vi "Object Tracking V2.vi"() -> ()   [LabVIEW 2012]
uses:
  <vilib>/userdefined/High Color/IMAQdx.ctl
  <vilib>/vision/Pattern Matching.llb/IMAQ Curve Parameters.ctl
  <vilib>/vision/driver/IMAQdx.llb/IMAQdx Buffer Number Mode.ctl
  <vilib>/vision/driver/NI_Vision_Acquisition_Software.lvlib
  <vilib>/vision/NI_Vision_Development_Module.lvlib
panel:
  in  "Match Type":enum16{"Geometric Matching", "Pattern Matching"}(ring)=enum."Pattern Matching"
  in  "Match":bool
  out "Matches":T1(array[cluster]) {"Bounding Box"."y" format="%.2f"; "Bounding Box"."x" format="%.2f"; "Position"."y" format="%.2f"; "Position"."x" format="%.2f"; "Score" format="%.2f"; "Scale" format="%.2f"; "Angle" format="%.2f"}
  in  "Learn":bool
  in  "Snap Frame":bool
  in  "Camera Name":T2="cam0"
  in  "Stop Button":bool
  in  "Geometric Match Mode":T3={"Rotation"=TRUE, "Scale"=FALSE, "Occlusion"=FALSE, "Reserved"=FALSE, "Reserved"=FALSE, "Reserved"=FALSE}
  in  "Pattern Match Mode":u16(ring)=1 items=["Shift Invariant", "Rotation Invariant"]
  in  "Minimum Score":sgl=600.0
  in  "Nb of Matches":i32=1
  in  "Subpixel Accuracy":bool
  in  "Minimum Contrast":i32=10
  in  "Curve Parameters":T4={"Extraction Mode"=0, "Edge Threshold"=75, "Edge Filter Size"=1, "Min Length"=25, "Row Search Step Size"=15, "Col Search Step Size"=15, "Max Endpoint Gap"=10, "Closed"=FALSE, "Subpixel"=FALSE} {"Extraction Mode" items=["Normal", "Uniform Regions"]; "Edge Filter Size" items=["Fine", "Normal", "Contour Tracing"]; "Max Endpoint Gap" min=0; "Col Search Step Size" min=1 max=255 step=1; "Row Search Step Size" min=1 max=255 step=1; "Min Length" min=0; "Edge Threshold" min=1 max=350 step=1}
  out "Template":T5(plugin-control)
  out "Snap Image":T5(plugin-control)
  out "Image Out":T5(plugin-control)
  # "1. Run the VI\n\n2. Click \"Snap Frame\" (make sure the object that you want to track\nit in the image at the time you snap the frame\n\n3. Use the mouse to select that object that you wish to track. This is done in the bottow left frame,\n\n4. Click \"Learn\" (This area is not saved at the new template image as seen in the bottom right frame)\n\n5. Click \"Match\" the program will then look for the template image and display the resutls with a red box."
  # "1."
  # "2."
  # "3."
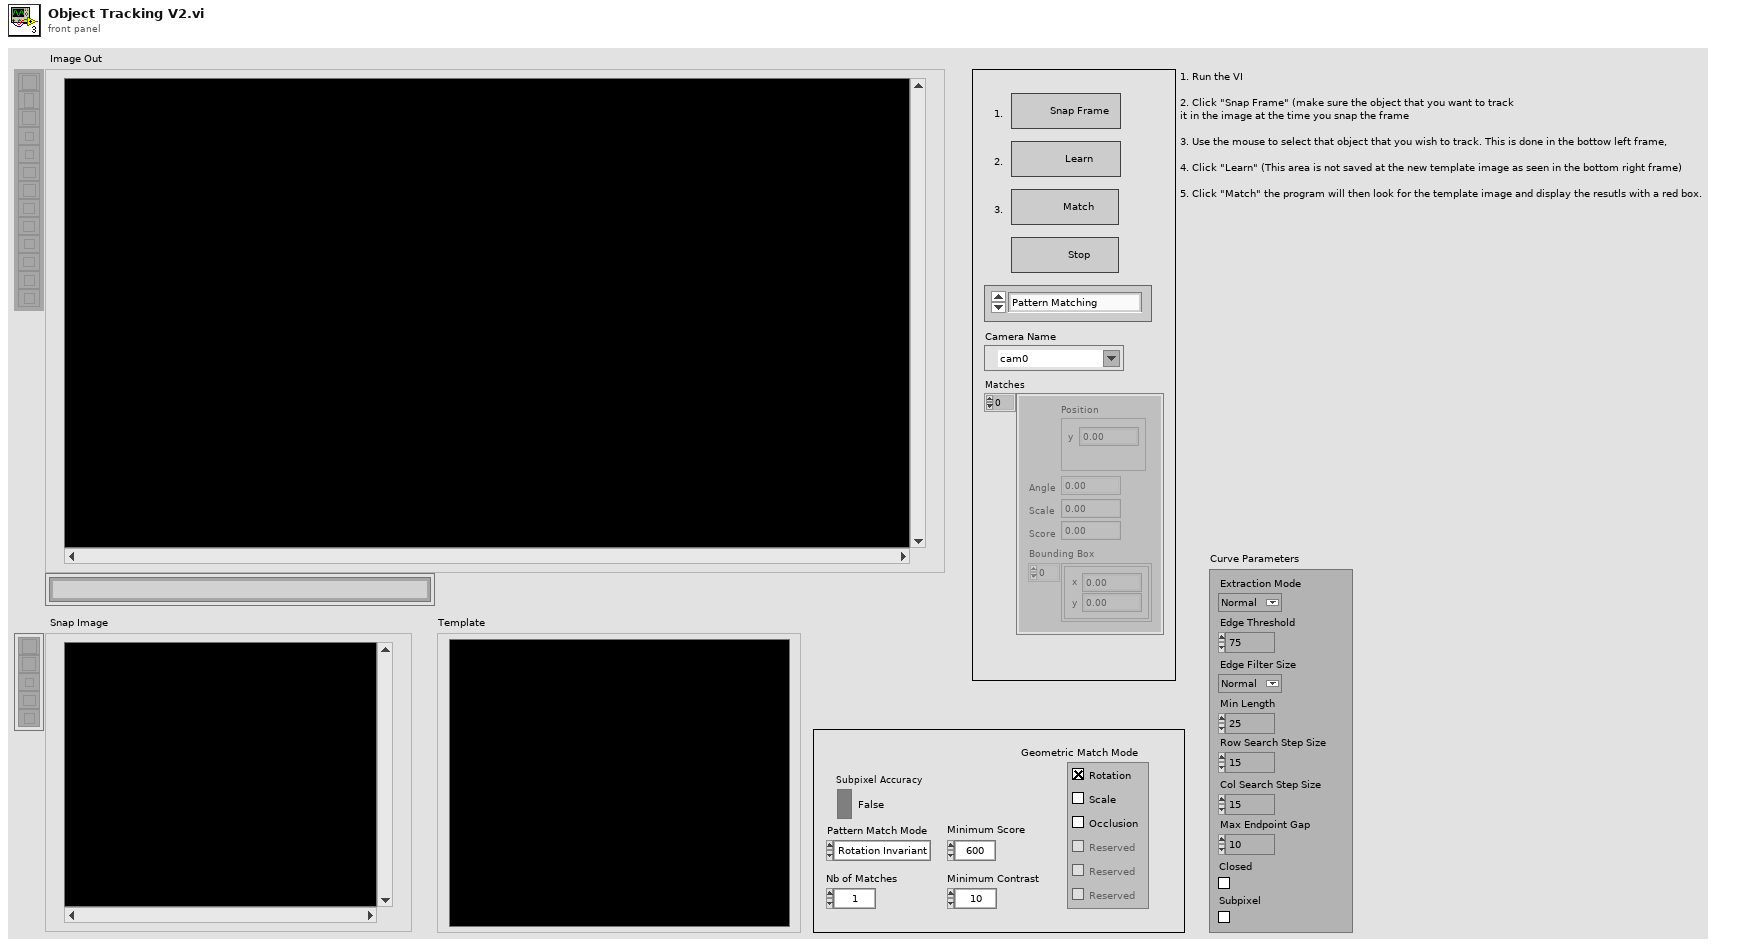
[diagram p1: front panel]
types:
  T1 = cluster{"Position":cluster{"x":sgl, "y":sgl}, "Angle":sgl, "Scale":sgl, "Score":sgl, "Bounding Box":cluster{"x":sgl, "y":sgl}[]}[]
  T2 = typedef "IMAQdx.ctl" = refnum<k21>
  T3 = cluster{"Rotation":bool, "Scale":bool, "Occlusion":bool, "Reserved":bool, "Reserved":bool, "Reserved":bool}
  T4 = typedef "IMAQ Curve Parameters.ctl" = cluster{"Extraction Mode":u32, "Edge Threshold":i32, "Edge Filter Size":u32, "Min Length":i32, "Row Search Step Size":i32, "Col Search Step Size":i32, "Max Endpoint Gap":i32, "Closed":bool, "Subpixel":bool}
  T5 = typedef "IMAQ Image.ctl" = refnum<image>
  T6 = cluster{"Global Rectangle":i32[], "Contours":cluster{"Contour Type":u32, "ROI Type":u32, "Points":i32[]}[]}
  T7 = typedef "NI_Vision_Acquisition_Software.lvlib/IMAQdx Buffer Number Mode.ctl" = enum32{"Next", "Last", "Buffer Number"}
  T8 = cluster{i32[], cluster{"Contour Type":u32, "ROI Type":u32, i32[]}[]}
  T9 = typedef "Image Type" = u32
  T10 = typedef "IMAQ GM Match Report.ctl" = cluster{"Position":cluster{"x":sgl, "y":sgl}, "Angle":sgl, "Scale":sgl, "Score":sgl, "Bounding Box":cluster{"x":sgl, "y":sgl}[], "Contrast Reversed":bool, "Occlusion %":sgl, "Template Target Curve Score":sgl, "Target Template Curve Score":sgl, "Correlation Score":sgl}
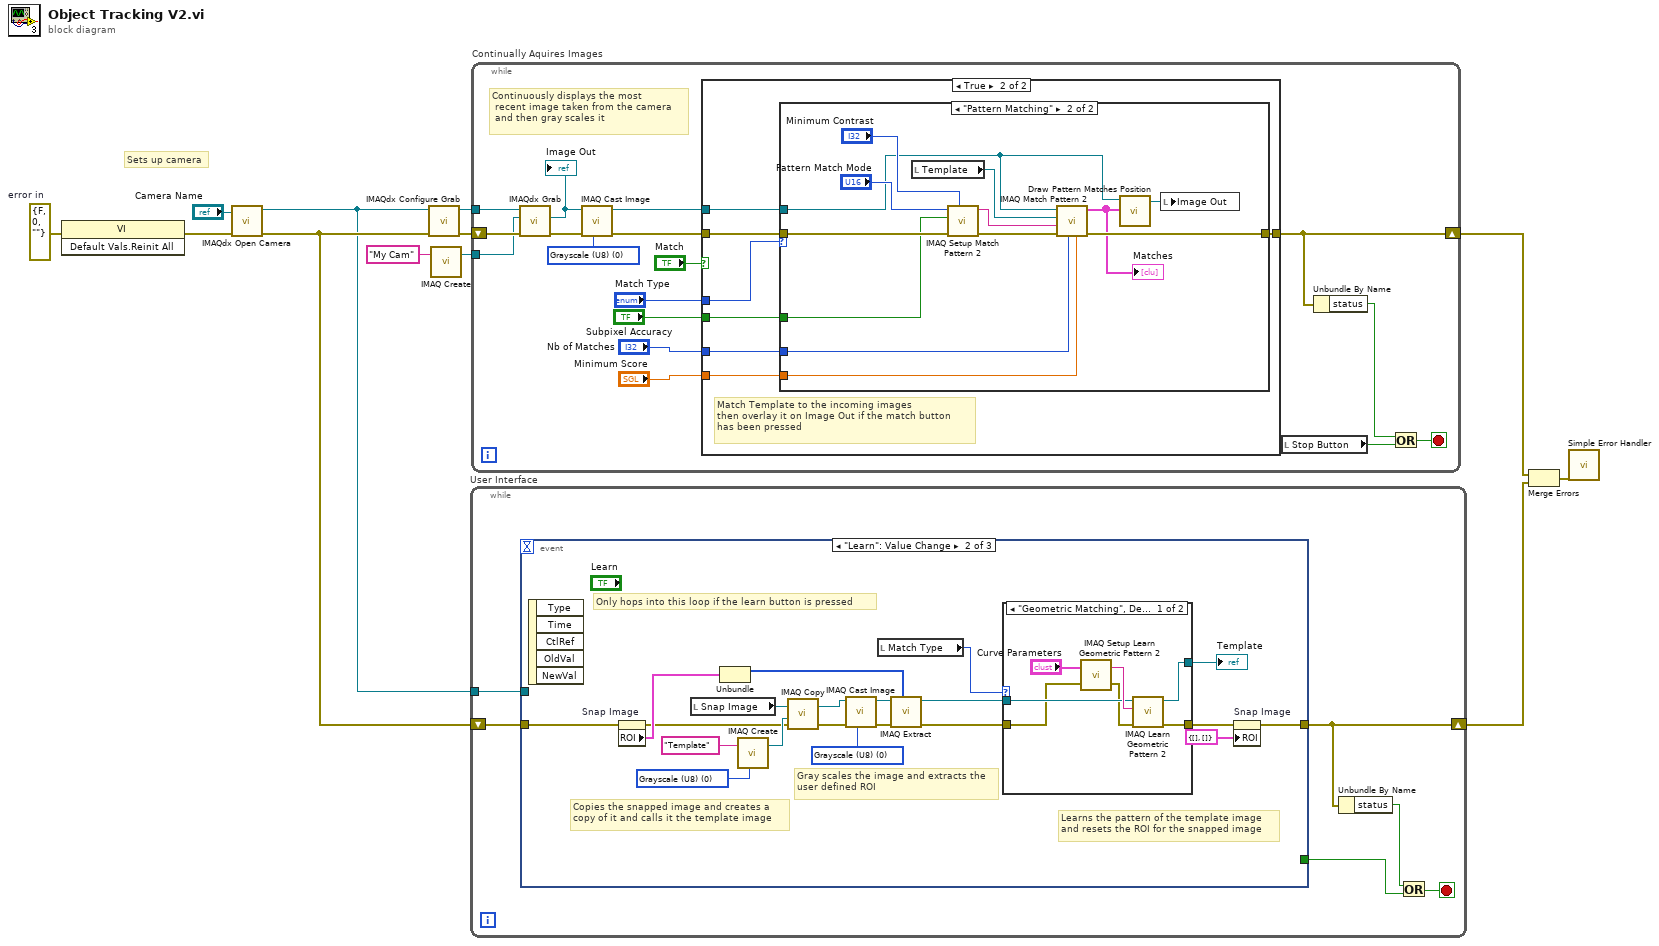
[diagram p0: block diagram]
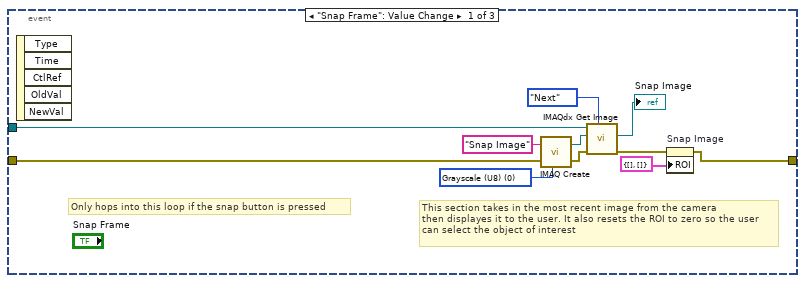
[diagram p2: hidden frame]
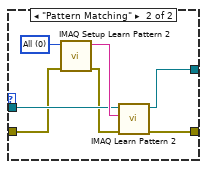
[diagram p3: hidden frame]
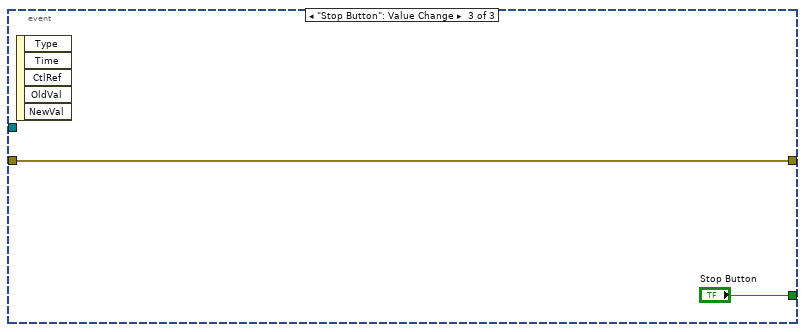
[diagram p4: hidden frame]
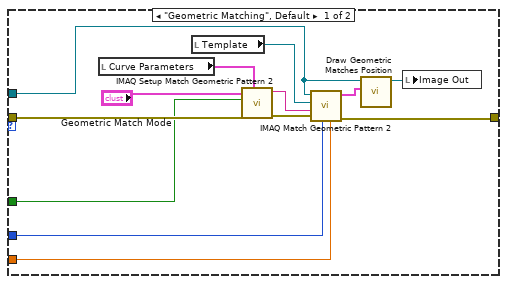
[diagram p6: hidden frame]
diagram:
  w9 = errorcluster {"status"=FALSE, "code"=0, "source"=""}  # error in
  # "Sets up camera"
  n1 = invoke class="VI" method="Default Vals.Reinit All"(error in=w9) -> (error out=w8:errorcluster)  [unwired: 2 in, 2 out]
  n2 = call <vilib>:"IMAQdx Open Camera.vi"("error in"=w8, "Session In"="Camera Name") -> ("error out"=w5:errorcluster, "Session Out"=w4:T2)  [unwired: 8 in]
  n3 = call <vilib>:"IMAQdx Configure Grab.vi"("error in"=w5, "Session In"=w4) -> ("error out"=w11:errorcluster, "Session Out"=w12:T2)  [unwired: 8 in]
  n4 = call "IMAQ Create"("Image Name"="My Cam") -> ("New Image"=w7:T5)  [unwired: 4 in, 1 out]
  n5 = while "User Interface" {
    tunnel: w4 -> [w17]
    shift-right: [w14] -> w1
    shift-left: w5 -> [w18]
    stop <- w16 stop-if-true
    n6 = event shown="[1] \"Learn\": Value Change" {
      selector: _ -> [_ _ _]
      dyn-events: _ -> [_ _ _]
      timeout: _ -> [_ _ _]
      tunnel: [_ _ "Stop Button"] -> w15
      tunnel: w18 -> [w24 w47 w64]
      tunnel: w17 -> [w23 _ _]
      tunnel: [w19 w43 w64] -> w14
      event "Snap Frame": Value Change {
        w22 = T9 0 items=["Grayscale (U8)", "Grayscale (I16)", "Grayscale (SGL)", "Complex (CSG)", "RGB (U32)", "HSL (U32)", "RGB (U64)", "Grayscale (U16)"] ("Image Type")
        # "Only hops into this loop if the snap button is pressed"
        # "This section takes in the most recent image from the camera \nthen displayes it to the user. It also resets the ROI to zero so the user\ncan select the object of interest"
        n7 = event-data() -> ()  [unwired: 1 in, 5 out]
        n8 = call "IMAQ Create"("Image Name"="Snap Image", "Image Type"=w22, "error in (no error)"=w24) -> ("New Image"=w27:T5, "error out"=w26:errorcluster)  [unwired: 2 in]
        n9 = call <vilib>:"IMAQdx Get Image.vi"("Buffer Number Mode (Next)"=IMAQdx_Buffer_Number_Mode."Next", "error in"=w26, "Image In"=w27, "Session In"=w23) -> ("error out"=w21:errorcluster, "Image Out"=→"Snap Image":T5)  [unwired: 4 in, 2 out]
        n10 = property on="Snap Image" class="ImageControl"(error in=w21, "ROI"=T6 {"Global Rectangle"=[], "Contours"=[]}) -> (error out=w19:errorcluster)  [unwired: 1 in, 1 out]
      }
      event "Learn": Value Change {
        w36 = T9 0 items=["Grayscale (U8)", "Grayscale (I16)", "Grayscale (SGL)", "Complex (CSG)", "RGB (U32)", "HSL (U32)", "RGB (U64)", "Grayscale (U16)"] ("Image Type")
        w37 = T9 0 items=["Grayscale (U8)", "Grayscale (I16)", "Grayscale (SGL)", "Complex (CSG)", "RGB (U32)", "HSL (U32)", "RGB (U64)", "Grayscale (U16)"] ("Image Type")
        # "Learns the pattern of the template image\nand resets the ROI for the snapped image"
        # "Gray scales the image and extracts the\nuser defined ROI"
        # "Copies the snapped image and creates a \ncopy of it and calls it the template image"
        # "Only hops into this loop if the learn button is pressed"
        n11 = event-data() -> ()  [unwired: 1 in, 5 out]
        n12 = property on="Snap Image" class="ImageControl"(error in=w47) -> (error out=w38:errorcluster, "ROI"=w46:T6)  [unwired: 1 in, 1 out]
        n13 = local read "Snap Image"() -> (w41:T5)
        n14 = Unbundle(w46) -> ("Global Rectangle"=w45:i32[])  [unwired: 1 out]
        n15 = call "IMAQ Create"("Image Name"="Template", "Image Type"=w37) -> ("New Image"=w40:T5)  [unwired: 3 in, 1 out]
        n16 = call "IMAQ Copy"("error in (no error)"=w38, "Image Dst"=w40, "Image Src"=w41) -> ("error out"=w33:errorcluster, "Image Dst Out"=w35:T5)  [unwired: 3 in]
        n17 = call "IMAQ Cast Image"("Image Type"=w36, "error in (no error)"=w33, "Image Src"=w35) -> ("error out"=w32:errorcluster, "Image Dst Out"=w34:T5)  [unwired: 7 in]
        n18 = local read "Match Type"() -> (w31:enum16{"Geometric Matching", "Pattern Matching"})
        n19 = call "IMAQ Extract"("Optional Rectangle"=w45, "error in (no error)"=w32, "Image Src"=w34) -> ("error out"=w30:errorcluster, "Image Dst Out"=w49:T5)  [unwired: 3 in, 4 out]
        n20 = case shown="\"Geometric Matching\", Default" w31 {
          tunnel: w49 -> [w52 w62]
          tunnel: [w53 w60] -> w48
          tunnel: [w54 w58] -> w44
          tunnel: w30 -> [w51 w57]
          frame "Geometric Matching", Default {
            n21 = call "IMAQ Setup Learn Geometric Pattern 2"("error in (no error)"=w51, "Curve Parameters"="Curve Parameters") -> ("error out"=w50:errorcluster, "Learn Geometric Pattern 2 Setup Data"=w55:string)
            n22 = call "IMAQ Learn Geometric Pattern 2"("error in (no error)"=w50, "Learn Geometric Pattern 2 Setup Data"=w55, "Template Image"=w52) -> ("error out"=w54:errorcluster, "Template Image Out"=w53:T5)  [unwired: 7 in]
          }
          frame "Pattern Matching" {
            w61 = u16 0 items=["All", "Shift Information", "Rotation Information"] ("Learn Mode")
            n23 = call "IMAQ Setup Learn Pattern 2"("error in (no error)"=w57, "Learn Mode"=w61) -> ("error out"=w59:errorcluster, "Learn Pattern Setup Data"=w63:string)  [unwired: 8 out]
            n24 = call "IMAQ Learn Pattern 2"("error in (no error)"=w59, "Learn Pattern Setup Data"=w63, "Image"=w62) -> ("error out"=w58:errorcluster, "Template Image Out"=w60:T5)  [unwired: 1 in, 6 out]
          }
        }
        "Template" <- w48
        n25 = property on="Snap Image" class="ImageControl"(error in=w44, "ROI"=T8 {[], []}) -> (error out=w43:errorcluster)  [unwired: 1 in, 1 out]
      }
      event "Stop Button": Value Change {
        n26 = event-data() -> ()  [unwired: 1 in, 5 out]
      }
    }
    n27 = Unbundle By Name(w14) -> ("status"=w13:bool)
    n28 = Or(x=w13, y=w15) -> (x .or. y?=w16:bool)
  }
  n29 = while "Continually Aquires Images" {
    tunnel: w12 -> [w82]
    tunnel: w7 -> [w80]
    shift-right: [w71] -> w2
    shift-left: w11 -> [w81]
    stop <- w72 stop-if-true
    w77 = T9 0 items=["Grayscale (U8)", "Grayscale (I16)", "Grayscale (SGL)", "Complex (CSG)", "RGB (U32)", "HSL (U32)", "RGB (U64)", "Grayscale (U16)"] ("Image Type")
    # "Continuously displays the most\n recent image taken from the camera\n and then gray scales it"
    n30 = call <vilib>:"IMAQdx Grab.vi"("error in"=w81, "Image In"=w80, "Session In"=w82) -> ("error out"=w78:errorcluster, "Image Out"=w79:T5)  [unwired: 5 in, 2 out]
    "Image Out" <- w79
    n31 = call "IMAQ Cast Image"("Image Type"=w77, "error in (no error)"=w78, "Image Src"=w79) -> ("error out"=w76:errorcluster, "Image Dst Out"=w75:T5)  [unwired: 7 in]
    n32 = case shown="True" "Match" {
      tunnel: w76 -> [w83 w90]
      tunnel: w75 -> [_ w89]
      tunnel: [w83 w88] -> w71
      tunnel: "Nb of Matches" -> [_ w87]
      tunnel: "Minimum Score" -> [_ w86]
      tunnel: "Subpixel Accuracy" -> [_ w85]
      tunnel: "Match Type" -> [_ w84]
      frame False {
      }
      frame True {
        # "Match Template to the incoming images \nthen overlay it on Image Out if the match button\nhas been pressed"
        n33 = case shown="\"Pattern Matching\"" w84 {
          tunnel: w90 -> [w96 w111]
          tunnel: w89 -> [w93 w105]
          tunnel: [w98 w110] -> w88
          tunnel: w87 -> [w95 w109]
          tunnel: w86 -> [w94 w108]
          tunnel: w85 -> [w92 w107]
          frame "Geometric Matching", Default {
            n34 = local read "Curve Parameters"() -> (w100:T4)
            n35 = local read "Template"() -> (w103:T5)
            n36 = call "IMAQ Setup Match Geometric Pattern 2"("Curve Parameters"=w100, "error in (no error)"=w96, "Subpixel Accuracy"=w92, "Match Mode"="Geometric Match Mode") -> ("error out"=w102:errorcluster, "Match Geometric Pattern 2 Setup Data"=w99:string)  [unwired: 6 in]
            n37 = call "IMAQ Match Geometric Pattern 2"("Minimum Match Score"=w94, "Number of Matches Requested"=w95, "error in (no error)"=w102, "Match Geometric Pattern 2 Setup Data"=w99, "Template Image"=w103, "Image"=w93) -> ("error out"=w98:errorcluster, "Matches (pixel)"=w91:T10[])  [unwired: 2 in, 2 out]
            n38 = call "Draw Geometric Matches Position .vi"("Matches (pixel)"=w91, "Image"=w93) -> ("Image Out"=w97:T5)  [unwired: 9 out]
            n39 = local write "Image Out"(w97) -> ()
          }
          frame "Pattern Matching" {
            n40 = local read "Template"() -> (w113:T5)
            n41 = call "IMAQ Setup Match Pattern 2"("Minimum Contrast"="Minimum Contrast", "error in (no error)"=w111, "Subpixel Accuracy"=w107, "Match Mode"="Pattern Match Mode") -> ("error out"=w112:errorcluster, "Match Pattern Setup Data"=w116:string)  [unwired: 1 in, 5 out]
            n42 = call "IMAQ Match Pattern 2"("Minimum Match Score"=w108, "Number of Matches Requested"=w109, "error in (no error)"=w112, "Match Pattern Setup Data"=w116, "Template Image"=w113, "Image"=w105) -> ("error out"=w110:errorcluster, "Matches"=w106:T1)  [unwired: 1 in, 3 out]
            "Matches" <- w106
            n43 = call "Draw Pattern Matches Position .vi"("Matches"=w106, "Image"=w105) -> ("Image Out"=w104:T5)  [unwired: 9 in]
            n44 = local write "Image Out"(w104) -> ()
          }
        }
      }
    }
    n45 = local read "Stop Button"() -> (w73:bool)
    n46 = Unbundle By Name(w71) -> ("status"=w70:bool)
    n47 = Or(x=w70, y=w73) -> (x .or. y?=w72:bool)
  }
  n48 = Merge Errors(w2, w1) -> (w3:errorcluster)
  n49 = call <vilib>:"Simple Error Handler.vi"("error in (no error)"=w3) -> ()  [unwired: 4 in, 5 out]
